vi "Write Message.vi"(8 "error in (no error)":errorcluster, 10 "Message":string, 11 "Assertion Result In":refnum<class "Assertion Result.lvclass">) -> (0 "error out":errorcluster, 3 "Assertion Result Out":refnum<class "Assertion Result.lvclass">)   [LabVIEW 2020, in "Assertion Result.lvclass"]
uses:
  Assertion Result.lvclass
  Assertion Result.lvclass/Assertion Result.ctl
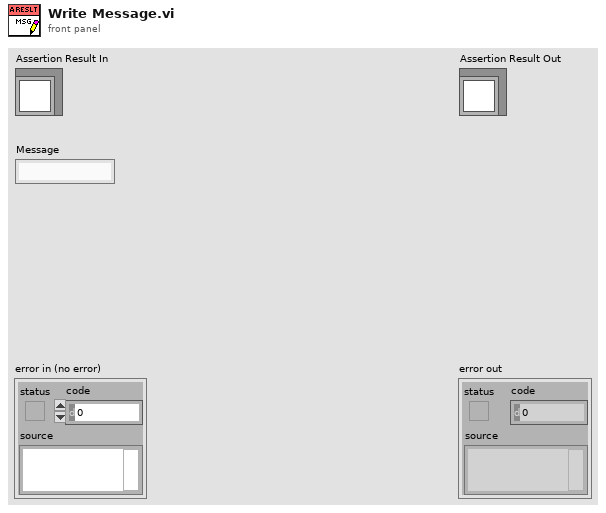
[diagram p1: front panel]
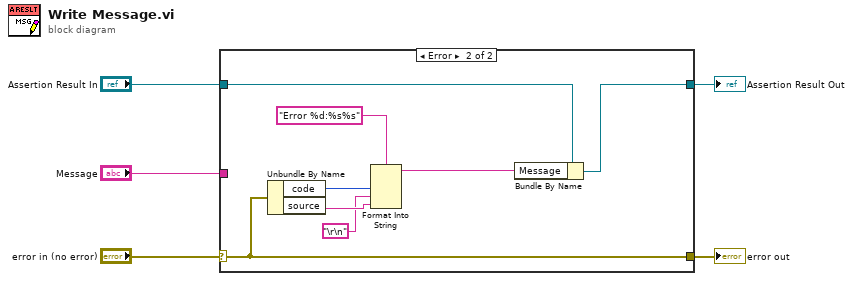
[diagram p0: block diagram]
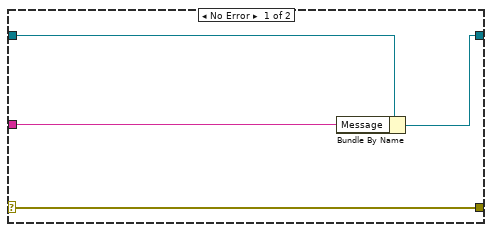
[diagram p2: hidden frame]
diagram:
  n1 = case shown="Error" "error in (no error)" {
    selector: "error in (no error)" -> [w9 w15]
    tunnel: [w9 w15] -> w4
    tunnel: [w7 w17] -> w2
    tunnel: "Assertion Result In" -> [w8 w16]
    tunnel: "Message" -> [w6 _]
    frame No Error {
      n2 = Bundle By Name(cluster=w8, "Message"=w6) -> (w7:refnum<class "Assertion Result.lvclass">)
    }
    frame Error {
      n3 = Unbundle By Name(w15) -> ("code"=w13:i32, "source"=w11:string)
      n4 = Format Into String(format string="Error %d:%s%s", w13, "\r\n", w11) -> (resulting string=w12:string)  [unwired: 2 in, 1 out]
      n5 = Bundle By Name(cluster=w16, "Message"=w12) -> (w17:refnum<class "Assertion Result.lvclass">)
    }
  }
  "error out" <- w4
  "Assertion Result Out" <- w2
